vi "Main.vi"() -> ()   [LabVIEW 2018] (continued)
            n437 = call "S7_Read.vi"("TCP"=w5185, "DB #"=u16 20, "读取长度"=u16 1, "寄存器类型"=w5227, "起始地址"=u32 0, "数据类型"=w5225, "error in"=w5184) -> ("TCP"=w5208:refnum<k5>, "数据"=w5222:u32[], "error out"=w5207:errorcluster)  [unwired: 5 in, 1 out]
            n438 = Index Array(array=w5222, index=0 ("索引")) -> (element=w5220:u32)
            n439 = Number To Boolean Array(number=w5220) -> (Boolean array=w5219:bool[])
            n440 = Index Array(array=w5219, index=2 ("索引")) -> (element=w5209:bool)
            "ST502扫码请求" <- w5209
            n441 = Unbundle By Name(w5187) -> ("扫码超时2"=w5200:string)
            n442 = Not Equal?(x=w5200, y="999") -> (x != y?=w5202:bool)
            n443 = Not(x=w5202) -> (.not. x?=w5203:bool)
            n444 = call <vilib>:"Boolean Crossing PtByPt.vi"("direction"=enum16{"either", "false-true", "true-false"}."false-true", "input"=w5209) -> ("crossing"=w5215:bool)  [unwired: 1 in]
            n445 = call <vilib>:"Boolean Crossing PtByPt.vi"("direction"=enum16{"either", "false-true", "true-false"}."true-false", "input"=w5209) -> ("crossing"=w5214:bool)  [unwired: 1 in]
            n446 = call "已用时间13"("Reset"=w5203) -> ("Time has Elapsed"=w5204:bool)  [unwired: 11 in, 7 out]
            n447 = Insert Into Array(array=bool[] [] ("数组"), index=0 ("索引"), new element #1=w5215, new element #2=w5214) -> (w5211:bool[])
            n448 = Boolean Array To Number(Boolean array=w5211) -> (number=w5210:u32)
            n449 = case shown="0, 默认" w5210 {
              tunnel: [cluster{"Data":string[], "State":T1} {"Data"=[], "State"=enum."读数据保存请求2"} ("元素") w5235 w5237] -> w5206
              tunnel: w5199 -> [_ w5236 w5238]
              frame 0, Default {
              }
              frame 1 {
                w5235 = cluster{"Data":string[], "State":T1} {"Data"=[], "State"=enum."读二维码2"} ("元素")
                n450 = Enqueue Element(queue=w5236, element=w5235, timeout in ms (-1)=10 ("超时毫秒(-1)")) -> ()  [unwired: 1 in, 3 out]
              }
              frame 2 {
                w5237 = cluster{"Data":string[], "State":T1} {"Data"=["999"], "State"=enum."扫码回复2"} ("元素")
                n451 = Enqueue Element(queue=w5238, element=w5237, timeout in ms (-1)=10 ("超时毫秒(-1)")) -> ()  [unwired: 1 in, 3 out]
              }
            }
            n452 = case shown="真" w5204 {
              tunnel: w5199 -> [_ w5231]
              frame False {
              }
              frame True {
                n453 = Enqueue Element(queue=w5231, element=cluster{"Data":string[], "State":T1} {"Data"=["999"], "State"=enum."扫码回复2"} ("元素"), timeout in ms (-1)=10 ("超时毫秒(-1)")) -> ()  [unwired: 1 in, 3 out]
              }
            }
          }
          frame "读二维码2" {
            w5255 = u16 0 items=["byte", "word", "Dword"] ("数据类型")
            w5252 = u8 132 items=["I/O (P)"=128, "Input (I)"=129, "Output (Q)"=130, "Bit Memory (M)"=131, "Data (DB)"=132, "Instance Data (DI)"=133, "Local Data (L)"=134, "Predecessor Local Data (VL)"=135] ("寄存器类型")
            n454 = call "S7_Read.vi"("TCP"=w5251, "DB #"=u16 20, "读取长度"=u16 17, "寄存器类型"=w5252, "起始地址"=u32 42, "数据类型"=w5255) -> ("TCP"=w5250:refnum<k5>, "数据"=w5256:u32[], "error out"=w5258:errorcluster)  [unwired: 6 in, 1 out]
            n455 = To Unsigned Word Integer(number=w5256) -> (unsigned 16bit integer=w5257:u16[])
            n456 = call "还原为字符串.vi"("error in (no error)"=w5258, "输入数组"=w5257) -> ("error out"=w5242:errorcluster, "字符串"=w5243:string)  [unwired: 8 in]
            n457 = Match Pattern(string=w5243, regular expression=" " ("正则表达式")) -> (before substring=w5240:string)  [unwired: 1 in, 3 out]
            n458 = flat-sequence {
              tunnel: w5242 -> [w5260]
              tunnel: [w5260] -> w5241
              tunnel: w5240 -> [w5259]
              tunnel: [w5262] -> w5247
              tunnel: w5241 -> [w5261]
              frame #0 {
                "503二维码" <- w5259
              }
              frame #1 {
                n459 = property on="ST503扫码请求(事件)" class="Bool (严格)"(error in=w5261, "Val(Sgnl)"=TRUE ("值(信号)")) -> (error out=w5262:errorcluster)  [unwired: 1 in, 1 out]
              }
            }
          }
          frame "扫码回复2" {
            n460 = Array Size(array=w5272) -> (size(s)=w5273:i32)
            n461 = case shown="3, 默认" w5273 {
              tunnel: w5272 -> [w5298 w5307]
              tunnel: w5271 -> [w5285 w5308]
              tunnel: [w5276 w5310] -> w5270
              tunnel: [w5275 w5309] -> w5269
              tunnel: [w5274 w5306] -> w5264
              frame 3, Default {
                w5288 = u8 132 items=["I/O (P)"=128, "Input (I)"=129, "Output (Q)"=130, "Bit Memory (M)"=131, "Data (DB)"=132, "Instance Data (DI)"=133, "Local Data (L)"=134, "Predecessor Local Data (VL)"=135] ("寄存器类型")
                w5287 = u16 1 items=["byte", "word", "Dword"] ("数据类型")
                w5295 = u8 132 items=["I/O (P)"=128, "Input (I)"=129, "Output (Q)"=130, "Bit Memory (M)"=131, "Data (DB)"=132, "Instance Data (DI)"=133, "Local Data (L)"=134, "Predecessor Local Data (VL)"=135] ("寄存器类型")
                w5296 = u16 1 items=["byte", "word", "Dword"] ("数据类型")
                w5302 = u8 132 items=["I/O (P)"=128, "Input (I)"=129, "Output (Q)"=130, "Bit Memory (M)"=131, "Data (DB)"=132, "Instance Data (DI)"=133, "Local Data (L)"=134, "Predecessor Local Data (VL)"=135] ("寄存器类型")
                w5301 = u16 1 items=["byte", "word", "Dword"] ("数据类型")
                n462 = Index Array(array=w5298) -> (element #1=w5274:string, element #2=w5281:string, element #3=w5280:string)  [unwired: 3 in]
                n463 = Equal?(x=w5280, y="OK") -> (x = y?=w5278:bool)
                n464 = Decimal String To Number(string=w5281, default (0L)=u32 0 ("默认(0 I32)")) -> (number=w5282:u32)  [unwired: 1 in, 1 out]
                n465 = case shown="假" w5278 {
                  tunnel: [u32 2 ("写入数据") u32 1 ("写入数据")] -> w5277
                  frame False {
                  }
                  frame True {
                  }
                }
                n466 = call "S7_Write.vi"("TCP"=w5285, "寄存器类型"=w5302, "DB #"=u16 20, "写入地址"=u32 18, "数据类型"=w5301, "写入数据"=w5282) -> ("TCP"=w5292:refnum<k5>, "error out"=w5293:errorcluster)  [unwired: 7 in, 1 out]
                n467 = call "S7_Write.vi"("TCP"=w5292, "寄存器类型"=w5295, "DB #"=u16 20, "写入地址"=u32 20, "数据类型"=w5296, "写入数据"=w5277, "error in"=w5293) -> ("TCP"=w5284:refnum<k5>, "error out"=w5283:errorcluster)  [unwired: 6 in, 1 out]
                n468 = Decimal String To Number(string=w5274, default (0L)=u32 0 ("默认(0 I32)")) -> (number=w5291:u32)  [unwired: 1 in, 1 out]
                n469 = call "S7_Write.vi"("TCP"=w5284, "寄存器类型"=w5288, "DB #"=u16 20, "写入地址"=u32 14, "数据类型"=w5287, "写入数据"=w5291, "error in"=w5283) -> ("TCP"=w5276:refnum<k5>, "error out"=w5275:errorcluster)  [unwired: 6 in, 1 out]
              }
              frame 1 {
                w5313 = u8 132 items=["I/O (P)"=128, "Input (I)"=129, "Output (Q)"=130, "Bit Memory (M)"=131, "Data (DB)"=132, "Instance Data (DI)"=133, "Local Data (L)"=134, "Predecessor Local Data (VL)"=135] ("寄存器类型")
                w5312 = u16 1 items=["byte", "word", "Dword"] ("数据类型")
                n470 = Index Array(array=w5307) -> (element=w5306:string)  [unwired: 1 in]
                n471 = Decimal String To Number(string=w5306, default (0L)=u32 0 ("默认(0 I32)")) -> (number=w5316:u32)  [unwired: 1 in, 1 out]
                n472 = call "S7_Write.vi"("TCP"=w5308, "寄存器类型"=w5313, "DB #"=u16 20, "写入地址"=u32 14, "数据类型"=w5312, "写入数据"=w5316) -> ("TCP"=w5310:refnum<k5>, "error out"=w5309:errorcluster)  [unwired: 7 in, 1 out]
              }
            }
            "扫码请求回复502" <- w5264
            n473 = Bundle By Name(cluster=w5266, "扫码超时2"=w5264) -> (w5265:T7)
          }
          frame "-- --------------" {
          }
          frame "读数据保存请求2" {
            w5350 = u16 0 items=["byte", "word", "Dword"] ("数据类型")
            w5352 = u8 132 items=["I/O (P)"=128, "Input (I)"=129, "Output (Q)"=130, "Bit Memory (M)"=131, "Data (DB)"=132, "Instance Data (DI)"=133, "Local Data (L)"=134, "Predecessor Local Data (VL)"=135] ("寄存器类型")
            n474 = call "S7_Read.vi"("TCP"=w5333, "DB #"=u16 20, "读取长度"=u16 1, "寄存器类型"=w5352, "起始地址"=u32 0, "数据类型"=w5350) -> ("TCP"=w5332:refnum<k5>, "数据"=w5347:u32[], "error out"=w5331:errorcluster)  [unwired: 6 in, 1 out]
            n475 = Index Array(array=w5347, index=0 ("索引")) -> (element=w5345:u32)
            n476 = Number To Boolean Array(number=w5345) -> (Boolean array=w5344:bool[])
            n477 = Unbundle By Name(w5323) -> ("数据保存超时2"=w5324:string)
            n478 = Index Array(array=w5344, index=3 ("索引")) -> (element=w5334:bool)
            "ST502数据读取" <- w5334
            n479 = Not Equal?(x=w5324, y="999") -> (x != y?=w5326:bool)
            n480 = Not(x=w5326) -> (.not. x?=w5327:bool)
            n481 = call <vilib>:"Boolean Crossing PtByPt.vi"("direction"=enum16{"either", "false-true", "true-false"}."false-true", "input"=w5334) -> ("crossing"=w5337:bool)  [unwired: 1 in]
            n482 = call <vilib>:"Boolean Crossing PtByPt.vi"("direction"=enum16{"either", "false-true", "true-false"}."true-false", "input"=w5334) -> ("crossing"=w5338:bool)  [unwired: 1 in]
            n483 = call "已用时间14"("Reset"=w5327) -> ("Time has Elapsed"=w5328:bool)  [unwired: 11 in, 7 out]
            n484 = Insert Into Array(array=bool[] [] ("数组"), index=0 ("索引"), new element #1=w5337, new element #2=w5338) -> (w5341:bool[])
            n485 = Boolean Array To Number(Boolean array=w5341) -> (number=w5342:u32)
            n486 = case shown="1" w5342 {
              tunnel: [cluster{"Data":string[], "State":T1} {"Data"=[], "State"=enum."看门狗"} ("元素") w5358 w5361] -> w5330
              tunnel: w5322 -> [_ w5359 w5362]
              frame 0, Default {
              }
              frame 1 {
                w5358 = cluster{"Data":string[], "State":T1} {"Data"=[], "State"=enum."读数据2"} ("元素")
                n487 = Enqueue Element(queue=w5359, element=w5358, timeout in ms (-1)=10 ("超时毫秒(-1)")) -> ()  [unwired: 1 in, 3 out]
              }
              frame 2 {
                w5361 = cluster{"Data":string[], "State":T1} {"Data"=["999"], "State"=enum."数据保存回复2"} ("元素")
                n488 = Enqueue Element(queue=w5362, element=w5361, timeout in ms (-1)=10 ("超时毫秒(-1)")) -> ()  [unwired: 1 in, 3 out]
              }
            }
            n489 = case shown="真" w5328 {
              tunnel: w5322 -> [_ w5354]
              frame False {
              }
              frame True {
                n490 = Enqueue Element(queue=w5354, element=cluster{"Data":string[], "State":T1} {"Data"=["999"], "State"=enum."数据保存回复2"} ("元素"), timeout in ms (-1)=10 ("超时毫秒(-1)")) -> ()  [unwired: 1 in, 3 out]
              }
            }
          }
          frame "读数据2" {
            w5373 = u16 1 items=["byte", "word", "Dword"] ("数据类型")
            w5377 = u8 132 items=["I/O (P)"=128, "Input (I)"=129, "Output (Q)"=130, "Bit Memory (M)"=131, "Data (DB)"=132, "Instance Data (DI)"=133, "Local Data (L)"=134, "Predecessor Local Data (VL)"=135] ("寄存器类型")
            n491 = call "S7_Read.vi"("TCP"=w5368, "DB #"=u16 20, "读取长度"=u16 1, "寄存器类型"=w5377, "起始地址"=u32 12, "数据类型"=w5373) -> ("TCP"=w5366:refnum<k5>, "数据"=w5372:u32[], "error out"=w5365:errorcluster)  [unwired: 6 in, 1 out]
            n492 = Index Array(array=w5372) -> (element=w5370:u32)  [unwired: 1 in]
            n493 = Equal?(x=w5370, y=u32 1) -> (x = y?=w5384:bool)
            n494 = case shown="假" w5384 {
              tunnel: ["NG" "OK"] -> w5367
              frame False {
              }
              frame True {
              }
            }
            n495 = Format Date/Time String(time format string (%c)="%Y-%m-%d" ("时间格式字符串(%c)")) -> (date/time string=w5379:string)  [unwired: 2 in]
            n496 = Get Date/Time String() -> (time string=w5378:string)  [unwired: 3 in, 1 out]
            n497 = Insert Into Array(array=string[] [] ("数组"), index=0 ("索引"), new element #1="503" ("新元素/子数组"), new element #2=w5367, new element #3=w5379, new element #4=w5378, new element #5=w5367) -> (w5363:string[])
            n498 = flat-sequence {
              tunnel: w5365 -> [w5389]
              tunnel: [w5389] -> w5364
              tunnel: w5363 -> [w5388]
              tunnel: [w5391] -> w5371
              tunnel: w5364 -> [w5390]
              frame #0 {
                "503读取数据" <- w5388
              }
              frame #1 {
                n499 = property on="ST503数据读取（事件）" class="Bool (严格)"(error in=w5390, "Val(Sgnl)"=TRUE ("值(信号)")) -> (error out=w5391:errorcluster)  [unwired: 1 in, 1 out]
              }
            }
          }
          frame "数据保存回复2" {
            w5408 = u8 132 items=["I/O (P)"=128, "Input (I)"=129, "Output (Q)"=130, "Bit Memory (M)"=131, "Data (DB)"=132, "Instance Data (DI)"=133, "Local Data (L)"=134, "Predecessor Local Data (VL)"=135] ("寄存器类型")
            w5409 = u16 1 items=["byte", "word", "Dword"] ("数据类型")
            n500 = Index Array(array=w5402, index=0 ("索引")) -> (element=w5395:string)
            "数据保存请求回复502" <- w5395
            n501 = Decimal String To Number(string=w5395, default (0L)=u32 0 ("默认(0 I32)")) -> (number=w5404:u32)  [unwired: 1 in, 1 out]
            n502 = call "S7_Write.vi"("TCP"=w5403, "寄存器类型"=w5408, "DB #"=u16 20, "写入地址"=u32 16, "数据类型"=w5409, "写入数据"=w5404) -> ("TCP"=w5401:refnum<k5>, "error out"=w5400:errorcluster)  [unwired: 7 in, 1 out]
            n503 = Bundle By Name(cluster=w5397, "数据保存超时2"=w5395) -> (w5396:T7)
          }
          frame "------------" {
          }
          frame "看门狗" {
            w5426 = "\r" ("正则表达式")
            w5435 = u16 0 items=["byte", "word", "Dword"] ("数据类型")
            w5437 = u8 132 items=["I/O (P)"=128, "Input (I)"=129, "Output (Q)"=130, "Bit Memory (M)"=131, "Data (DB)"=132, "Instance Data (DI)"=133, "Local Data (L)"=134, "Predecessor Local Data (VL)"=135] ("寄存器类型")
            w5458 = u8 132 items=["I/O (P)"=128, "Input (I)"=129, "Output (Q)"=130, "Bit Memory (M)"=131, "Data (DB)"=132, "Instance Data (DI)"=133, "Local Data (L)"=134, "Predecessor Local Data (VL)"=135] ("寄存器类型")
            w5457 = u16 1 items=["byte", "word", "Dword"] ("数据类型")
            n504 = Unbundle By Name(w5446) -> ("看门狗"=w5455:string)
            n505 = Decimal String To Number(string=w5455) -> (number=w5454:i32)  [unwired: 2 in, 1 out]
            n506 = Equal?(x=w5454, y=0) -> (x = y?=w5452:bool)
            n507 = case shown="假" w5452 {
              tunnel: [0 ("y") 1 ("y")] -> w5447
              frame False {
              }
              frame True {
              }
            }
            "50" <- w5447
            n508 = call "S7_Write.vi"("TCP"=w5451, "寄存器类型"=w5458, "DB #"=u16 20, "写入地址"=u32 22, "数据类型"=w5457, "写入数据"=w5447) -> ("TCP"=w5433:refnum<k5>, "error out"=w5432:errorcluster)  [unwired: 7 in, 1 out]
            n509 = Number To Decimal String(number=w5447) -> (decimal integer string=w5448:string)  [unwired: 1 in]
            n510 = Bundle By Name(cluster=w5446, "看门狗"=w5448) -> (w5445:T7)
            n511 = call "S7_Read.vi"("TCP"=w5433, "DB #"=u16 20, "读取长度"=u16 100, "寄存器类型"=w5437, "起始地址"=u32 60, "数据类型"=w5435, "error in"=w5432) -> ("TCP"=w5421:refnum<k5>, "数据"=w5443:u32[], "error out"=w5419:errorcluster)  [unwired: 5 in, 1 out]
            n512 = To Unsigned Word Integer(number=w5443) -> (unsigned 16bit integer=w5444:u16[])
            n513 = call "还原为字符串.vi"("输入数组"=w5444) -> ("字符串"=w5442:string)  [unwired: 9 in, 1 out]
            n514 = for {
              N: 5 -> [_]
              tunnel: w5442 -> [w5478]
              tunnel: [w5477] -> w5434 mode=indexing
              shift-right: [w5473] -> _
              shift-left: 0 ("长度（剩余）") -> [w5475]
              n515 = String Subset(string=w5478, offset (0)=w5475, length (rest)=20 ("长度（剩余）")) -> (substring=w5477:string)
              n516 = Add(x=w5475, y=20) -> (x+y=w5473:i32)
            }
            n517 = Index Array(array=w5434) -> (element #1=w5431:string, element #2=w5430:string, element #3=w5429:string, element #4=w5428:string, element #5=w5427:string)  [unwired: 5 in]
            n518 = Match Pattern(string=w5431, regular expression=w5426) -> (before substring=w5417:string)  [unwired: 1 in, 3 out]
            n519 = Match Pattern(string=w5430, regular expression=w5426) -> (before substring=→"ST502 Form Seal 5026860":string)  [unwired: 1 in, 3 out]
            n520 = Match Pattern(string=w5429, regular expression=w5426) -> (before substring=→"ST502 Support Ring 5027083":string)  [unwired: 1 in, 3 out]
            n521 = Match Pattern(string=w5428, regular expression=w5426) -> (before substring=→"ST502 O-Ring M0104976":string)  [unwired: 1 in, 3 out]
            n522 = Match Pattern(string=w5427, regular expression=w5426) -> (before substring=→"ST502 Pressure Plate M0105053":string)  [unwired: 1 in, 3 out]
            n523 = disable-structure shown="启用" {
              disable-tunnel: w5421 -> [w5462 w5466]
              disable-tunnel: [w5462 w5469] -> w5420
              disable-tunnel: w5419 -> [w5463 w5467]
              disable-tunnel: [w5463 w5468] -> w5418
              frame Disabled {
              }
              frame Enabled {
                w5471 = u8 132 items=["I/O (P)"=128, "Input (I)"=129, "Output (Q)"=130, "Bit Memory (M)"=131, "Data (DB)"=132, "Instance Data (DI)"=133, "Local Data (L)"=134, "Predecessor Local Data (VL)"=135] ("寄存器类型")
                w5465 = u16 1 items=["byte", "word", "Dword"] ("数据类型")
                n524 = local read "80产品型号"() -> (w5464:u32)
                n525 = call "S7_Write.vi"("TCP"=w5466, "寄存器类型"=w5471, "DB #"=u16 20, "写入地址"=u32 188, "数据类型"=w5465, "写入数据"=w5464, "error in"=w5467) -> ("TCP"=w5469:refnum<k5>, "error out"=w5468:errorcluster)  [unwired: 6 in, 1 out]
              }
            }
            n526 = disable-structure shown="启用" {
              disable-tunnel: w5417 -> [w5460 _]
              disable-tunnel: [w5460 "20181017/148"] -> w5416
              frame Disabled {
              }
              frame Enabled {
              }
            }
            "ST40 Circlip 5026621" <- w5416
          }
        }
      }
      n527 = while {
        shift-right: [w5486] -> _
        shift-left: cluster{"Data":string[], "State":T1} {"Data"=[], "State"=enum."PLC通讯初始化"} ("元素") -> [w5487]
        shift-right: [w5495] -> _
        shift-left: w133 -> [w5492]
        shift-right: [w5496] -> _
        shift-left: _ -> [w5493]
        tunnel: w115 -> [w5488]
        tunnel: w114 -> [w5483]
        tunnel: w132 -> [_]
        shift-right: [w5482] -> _
        shift-left: _ -> [w5481]
        stop <- w5484 stop-if-true
        # "OP60"
        n528 = local read "退出"() -> (w5491:bool)
        n529 = Wait (ms)(milliseconds to wait=u32 20 ("等待时间（毫秒）")) -> ()  [unwired: 1 out]
        n530 = call "状态判断.vi"("error IO"=w5492, "退出？"=w5491, "簇 输入"=w5487, "队列输入"=w5488) -> ("簇"=w5490:cluster{"Data":string[], "State":T1})  [unwired: 6 in, 1 out]
        n531 = Unbundle By Name(w5490) -> ("Data"=w5485:string[], "State"=w5489:T1)
        "60_State" <- w5489
        n532 = case shown="\"看门狗\"" w5489 {
          tunnel: [w5504 w5545 w5567 w5598 w5619 w5670 w5690 w5722 w5749 w5764 refnum<k5> refnum ("TCP") refnum<k5> refnum ("TCP") w5786 w5811 w5852 w5873 w5924 w5935 w5975 w6005 w6014] -> w5496
          tunnel: [w5503 errorcluster {"status"=FALSE, "code"=0, "source"=""} ("error out") w5566 w5594 w5618 errorcluster {"status"=FALSE, "code"=0, "source"=""} ("error out") w5689 w5712 w5750 errorcluster {"status"=FALSE, "code"=0, "source"=""} ("error out") errorcluster {"status"=FALSE, "code"=0, "source"=""} ("error out") w5776 errorcluster {"status"=FALSE, "code"=0, "source"=""} ("error out") w5808 w5851 w5872 errorcluster {"status"=FALSE, "code"=0, "source"=""} ("error out") w5934 w5974 w6004 w6016] -> w5495
          tunnel: w5493 -> [_ w5545 w5568 w5599 w5620 w5670 w5691 w5736 w5752 w5764 w5770 w5777 w5786 w5792 w5853 w5874 w5924 w5936 w5970 w6006 w6046]
          tunnel: w5488 -> [w5531 _ w5548 _ _ _ w5671 _ _ _ w5766 w5778 _ w5802 _ _ _ w5925 _ _ _]
          tunnel: [cluster{"Data":string[], "State":T1} {"Data"=[], "State"=enum."读扫码请求"} ("元素") cluster{"Data":string[], "State":T1} {"Data"=[], "State"=enum."读扫码请求"} ("元素") w5556 cluster{"Data":string[], "State":T1} {"Data"=[], "State"=enum."读数据保存请求"} ("元素") cluster{"Data":string[], "State":T1} {"Data"=[], "State"=enum."读数据保存请求"} ("元素") cluster{"Data":string[], "State":T1} {"Data"=[], "State"=enum."读数据保存请求"} ("元素") w5679 cluster{"Data":string[], "State":T1} {"Data"=[], "State"=enum."读扫码请求2"} ("元素") cluster{"Data":string[], "State":T1} {"Data"=[], "State"=enum."读扫码请求2"} ("元素") cluster{"Data":string[], "State":T1} {"Data"=[], "State"=enum."读扫码请求2"} ("元素") cluster{"Data":string[], "State":T1} {"Data"=[], "State"=enum."PLC通讯初始化"} ("元素") cluster{"Data":string[], "State":T1} {"Data"=[], "State"=enum."退出"} ("元素") cluster{"Data":string[], "State":T1} {"Data"=[], "State"=enum."读扫码请求2"} ("元素") w5810 cluster{"Data":string[], "State":T1} {"Data"=[], "State"=enum."读数据保存请求2"} ("元素") cluster{"Data":string[], "State":T1} {"Data"=[], "State"=enum."读数据保存请求2"} ("元素") cluster{"Data":string[], "State":T1} {"Data"=[], "State"=enum."读数据保存请求2"} ("元素") w5933 cluster{"Data":string[], "State":T1} {"Data"=[], "State"=enum."看门狗"} ("元素") cluster{"Data":string[], "State":T1} {"Data"=[], "State"=enum."看门狗"} ("元素") cluster{"Data":string[], "State":T1} {"Data"=[], "State"=enum."读扫码请求"} ("元素")] -> w5486
          tunnel: w5485 -> [_ _ _ _ w5616 _ _ _ w5751 _ _ _ _ _ _ w5875 _ _ _ w6003 _]
          tunnel: [FALSE FALSE FALSE FALSE FALSE FALSE FALSE FALSE FALSE FALSE FALSE TRUE FALSE FALSE FALSE FALSE FALSE FALSE FALSE FALSE FALSE] -> w5484
          tunnel: w5483 -> [_ _ _ _ _ _ _ w5729 _ _ w5767 w5779 _ _ _ _ _ _ _ _ _]
          tunnel: [T9 {"扫码超时1"="999", "数据保存超时1"="999", "扫码超时2"="999", "数据保存超时2"="999", "看门狗"="999"} w5541 w5549 w5595 w5614 w5666 w5672 w5719 w5745 w5760 w5765 w5774 w5782 w5790 w5848 w5868 w5920 w5926 w5971 w5998 w6040] -> w5482
          tunnel: w5481 -> [_ w5541 w5549 w5595 w5615 w5666 w5672 w5719 w5746 w5760 w5765 w5774 w5782 w5791 w5848 w5869 w5920 w5926 w5971 w6000 w6041]
          frame "PLC通讯初始化", Default {
            w5516 = u16 0 items=["byte", "word", "Dword"] ("数据类型")
            w5520 = u8 132 items=["I/O (P)"=128, "Input (I)"=129, "Output (Q)"=130, "Bit Memory (M)"=131, "Data (DB)"=132, "Instance Data (DI)"=133, "Local Data (L)"=134, "Predecessor Local Data (VL)"=135] ("寄存器类型")
            w5509 = u16 0 items=["byte", "word", "Dword"] ("数据类型")
            w5513 = u8 132 items=["I/O (P)"=128, "Input (I)"=129, "Output (Q)"=130, "Bit Memory (M)"=131, "Data (DB)"=132, "Instance Data (DI)"=133, "Local Data (L)"=134, "Predecessor Local Data (VL)"=135] ("寄存器类型")
            w5539 = u8 0 items=["S7-1200.200.200SMART"=0, "S7-300"=2, "S7-400"=3] ("PLC 系列")
            n533 = call "S7_Open.vi"("IP 地址"="192.168.0.60", "PLC 系列"=w5539, "超时（MS）"=100) -> ("TCP"=w5506:refnum<k5>, "error out"=w5505:errorcluster)  [unwired: 10 in, 1 out]
            n534 = Unbundle By Name(w5505) -> ("status"=→"ST60通讯状态":bool)
            n535 = Enqueue Element(queue=w5531, element=cluster{"Data":string[], "State":T1} {"Data"=["999"], "State"=enum."扫码回复"} ("元素")) -> (queue out=w5535:refnum<queue>, error out=w5534:errorcluster)  [unwired: 2 in, 1 out]
            n536 = call "S7_Read.vi"("TCP"=w5506, "DB #"=u16 20, "读取长度"=u16 17, "寄存器类型"=w5513, "起始地址"=u32 24, "数据类型"=w5509, "error in"=w5505) -> ("TCP"=w5521:refnum<k5>, "数据"=w5508:u32[], "error out"=w5522:errorcluster)  [unwired: 5 in, 1 out]
            n537 = To Unsigned Word Integer(number=w5508) -> (unsigned 16bit integer=w5507:u16[])
            n538 = call "还原为字符串.vi"("输入数组"=w5507) -> ("字符串"=w5501:string)  [unwired: 9 in, 1 out]
            n539 = Enqueue Element(queue=w5535, element=cluster{"Data":string[], "State":T1} {"Data"=["999"], "State"=enum."数据保存回复"} ("元素"), error in (no error)=w5534) -> (queue out=w5524:refnum<queue>, error out=w5523:errorcluster)  [unwired: 1 in, 1 out]
            n540 = Match Pattern(string=w5501, regular expression=" " ("正则表达式")) -> (before substring=w5500:string)  [unwired: 1 in, 3 out]
            n541 = local write "601二维码"(w5500) -> ()
            n542 = Enqueue Element(queue=w5524, element=cluster{"Data":string[], "State":T1} {"Data"=["999"], "State"=enum."扫码回复2"} ("元素"), error in (no error)=w5523) -> (queue out=w5527:refnum<queue>, error out=w5528:errorcluster)  [unwired: 1 in, 1 out]
            n543 = call "S7_Read.vi"("TCP"=w5521, "DB #"=u16 20, "读取长度"=u16 17, "寄存器类型"=w5520, "起始地址"=u32 42, "数据类型"=w5516, "error in"=w5522) -> ("TCP"=w5504:refnum<k5>, "数据"=w5515:u32[], "error out"=w5503:errorcluster)  [unwired: 5 in, 1 out]
            n544 = Enqueue Element(queue=w5527, element=cluster{"Data":string[], "State":T1} {"Data"=["999"], "State"=enum."数据保存回复2"} ("元素"), error in (no error)=w5528) -> ()  [unwired: 1 in, 3 out]
            n545 = To Unsigned Word Integer(number=w5515) -> (unsigned 16bit integer=w5514:u16[])
            n546 = call "还原为字符串.vi"("输入数组"=w5514) -> ("字符串"=w5498:string)  [unwired: 9 in, 1 out]
            n547 = Match Pattern(string=w5498, regular expression=" " ("正则表达式")) -> (before substring=w5497:string)  [unwired: 1 in, 3 out]
            n548 = local write "602二维码"(w5497) -> ()
          }
          frame "--------------" {
          }
          frame "读扫码请求" {
            w5576 = u16 0 items=["byte", "word", "Dword"] ("数据类型")
            w5578 = u8 132 items=["I/O (P)"=128, "Input (I)"=129, "Output (Q)"=130, "Bit Memory (M)"=131, "Data (DB)"=132, "Instance Data (DI)"=133, "Local Data (L)"=134, "Predecessor Local Data (VL)"=135] ("寄存器类型")
            n549 = call "S7_Read.vi"("TCP"=w5568, "DB #"=u16 20, "读取长度"=u16 1, "寄存器类型"=w5578, "起始地址"=u32 0, "数据类型"=w5576) -> ("TCP"=w5567:refnum<k5>, "数据"=w5573:u32[], "读取成功"=w5546:bool, "error out"=w5566:errorcluster)  [unwired: 6 in]
            n550 = Not(x=w5546) -> (.not. x?=w5547:bool)
            n551 = local write "ST60通讯状态"(w5547) -> ()
            n552 = Index Array(array=w5573, index=0 ("索引")) -> (element=w5571:u32)
            n553 = Number To Boolean Array(number=w5571) -> (Boolean array=w5570:bool[])
            n554 = Index Array(array=w5570, index=0 ("索引")) -> (element=w5555:bool)
            "ST601扫码请求" <- w5555
            n555 = Unbundle By Name(w5549) -> ("扫码超时1"=w5550:string)
            n556 = Not Equal?(x=w5550, y="999") -> (x != y?=w5552:bool)
            n557 = Not(x=w5552) -> (.not. x?=w5553:bool)
            n558 = call <vilib>:"Boolean Crossing PtByPt.vi"("direction"=enum16{"either", "false-true", "true-false"}."false-true", "input"=w5555) -> ("crossing"=w5562:bool)  [unwired: 1 in]
            n559 = call <vilib>:"Boolean Crossing PtByPt.vi"("direction"=enum16{"either", "false-true", "true-false"}."true-false", "input"=w5555) -> ("crossing"=w5561:bool)  [unwired: 1 in]
            n560 = call "已用时间17"("Reset"=w5553) -> ("Time has Elapsed"=w5554:bool)  [unwired: 11 in, 7 out]
            n561 = Insert Into Array(array=bool[] [] ("数组"), index=0 ("索引"), new element #1=w5562, new element #2=w5561) -> (w5558:bool[])
            n562 = Boolean Array To Number(Boolean array=w5558) -> (number=w5557:u32)
            n563 = case shown="2" w5557 {
              tunnel: [cluster{"Data":string[], "State":T1} {"Data"=[], "State"=enum."读数据保存请求"} ("元素") w5584 w5587] -> w5556
              tunnel: w5548 -> [_ w5585 w5588]
              frame 0, Default {
              }
              frame 1 {
                w5584 = cluster{"Data":string[], "State":T1} {"Data"=[], "State"=enum."读二维码"} ("元素")
                n564 = Enqueue Element(queue=w5585, element=w5584, timeout in ms (-1)=10 ("超时毫秒(-1)")) -> ()  [unwired: 1 in, 3 out]
              }
              frame 2 {
                w5587 = cluster{"Data":string[], "State":T1} {"Data"=["999"], "State"=enum."扫码回复"} ("元素")
                n565 = Enqueue Element(queue=w5588, element=w5587, timeout in ms (-1)=10 ("超时毫秒(-1)")) -> ()  [unwired: 1 in, 3 out]
              }
            }
            n566 = case shown="真" w5554 {
              tunnel: w5548 -> [_ w5580]
              frame False {
              }
              frame True {
                n567 = Enqueue Element(queue=w5580, element=cluster{"Data":string[], "State":T1} {"Data"=["999"], "State"=enum."扫码回复"} ("元素"), timeout in ms (-1)=10 ("超时毫秒(-1)")) -> ()  [unwired: 1 in, 3 out]
              }
            }
          }
          frame "读二维码" {
            w5604 = u16 0 items=["byte", "word", "Dword"] ("数据类型")
            w5600 = u8 132 items=["I/O (P)"=128, "Input (I)"=129, "Output (Q)"=130, "Bit Memory (M)"=131, "Data (DB)"=132, "Instance Data (DI)"=133, "Local Data (L)"=134, "Predecessor Local Data (VL)"=135] ("寄存器类型")
            n568 = call "S7_Read.vi"("TCP"=w5599, "DB #"=u16 20, "读取长度"=u16 17, "寄存器类型"=w5600, "起始地址"=u32 24, "数据类型"=w5604) -> ("TCP"=w5598:refnum<k5>, "数据"=w5605:u32[], "error out"=w5607:errorcluster)  [unwired: 6 in, 1 out]
            n569 = To Unsigned Word Integer(number=w5605) -> (unsigned 16bit integer=w5606:u16[])
            n570 = call "还原为字符串.vi"("error in (no error)"=w5607, "输入数组"=w5606) -> ("error out"=w5591:errorcluster, "字符串"=w5592:string)  [unwired: 8 in]
            n571 = Match Pattern(string=w5592, regular expression=" " ("正则表达式")) -> (before substring=w5589:string)  [unwired: 1 in, 3 out]
            n572 = flat-sequence {
              tunnel: w5591 -> [w5609]
              tunnel: [w5609] -> w5590
              tunnel: w5589 -> [w5608]
              tunnel: [w5611] -> w5594
              tunnel: w5590 -> [w5610]
              frame #0 {
                "601二维码" <- w5608
              }
              frame #1 {
                n573 = property on="ST601扫码请求(事件)" class="Bool (严格)"(error in=w5610, "Val(Sgnl)"=TRUE ("值(信号)")) -> (error out=w5611:errorcluster)  [unwired: 1 in, 1 out]
              }
            }
          }
          frame "扫码回复" {
            n574 = Array Size(array=w5616) -> (size(s)=w5617:i32)
            n575 = case shown="3, 默认" w5617 {
              tunnel: w5616 -> [w5624 w5658]
              tunnel: w5620 -> [w5625 w5645]
              tunnel: [w5627 w5636] -> w5619
              tunnel: [w5626 w5635] -> w5618
              tunnel: [w5623 w5634] -> w5613
              frame 1 {
                w5630 = u8 132 items=["I/O (P)"=128, "Input (I)"=129, "Output (Q)"=130, "Bit Memory (M)"=131, "Data (DB)"=132, "Instance Data (DI)"=133, "Local Data (L)"=134, "Predecessor Local Data (VL)"=135] ("寄存器类型")
                w5629 = u16 1 items=["byte", "word", "Dword"] ("数据类型")
                n576 = Index Array(array=w5624) -> (element=w5623:string)  [unwired: 1 in]
                n577 = Decimal String To Number(string=w5623, default (0L)=u32 0 ("默认(0 I32)")) -> (number=w5633:u32)  [unwired: 1 in, 1 out]
                n578 = call "S7_Write.vi"("TCP"=w5625, "寄存器类型"=w5630, "DB #"=u16 20, "写入地址"=u32 2, "数据类型"=w5629, "写入数据"=w5633) -> ("TCP"=w5627:refnum<k5>, "error out"=w5626:errorcluster)  [unwired: 7 in, 1 out]
              }
              frame 3, Default {
                w5648 = u8 132 items=["I/O (P)"=128, "Input (I)"=129, "Output (Q)"=130, "Bit Memory (M)"=131, "Data (DB)"=132, "Instance Data (DI)"=133, "Local Data (L)"=134, "Predecessor Local Data (VL)"=135] ("寄存器类型")
                w5647 = u16 1 items=["byte", "word", "Dword"] ("数据类型")
                w5655 = u8 132 items=["I/O (P)"=128, "Input (I)"=129, "Output (Q)"=130, "Bit Memory (M)"=131, "Data (DB)"=132, "Instance Data (DI)"=133, "Local Data (L)"=134, "Predecessor Local Data (VL)"=135] ("寄存器类型")
                w5656 = u16 1 items=["byte", "word", "Dword"] ("数据类型")
                w5662 = u8 132 items=["I/O (P)"=128, "Input (I)"=129, "Output (Q)"=130, "Bit Memory (M)"=131, "Data (DB)"=132, "Instance Data (DI)"=133, "Local Data (L)"=134, "Predecessor Local Data (VL)"=135] ("寄存器类型")
                w5661 = u16 1 items=["byte", "word", "Dword"] ("数据类型")
                n579 = Index Array(array=w5658) -> (element #1=w5634:string, element #2=w5641:string, element #3=w5640:string)  [unwired: 3 in]
                n580 = Equal?(x=w5640, y="OK") -> (x = y?=w5638:bool)
                n581 = Decimal String To Number(string=w5641, default (0L)=u32 0 ("默认(0 I32)")) -> (number=w5642:u32)  [unwired: 1 in, 1 out]
                n582 = case shown="假" w5638 {
                  tunnel: [u32 2 ("写入数据") u32 1 ("写入数据")] -> w5637
                  frame False {
                  }
                  frame True {
                  }
                }
                n583 = call "S7_Write.vi"("TCP"=w5645, "寄存器类型"=w5662, "DB #"=u16 20, "写入地址"=u32 8, "数据类型"=w5661, "写入数据"=w5642) -> ("TCP"=w5652:refnum<k5>, "error out"=w5653:errorcluster)  [unwired: 7 in, 1 out]
                n584 = call "S7_Write.vi"("TCP"=w5652, "寄存器类型"=w5655, "DB #"=u16 20, "写入地址"=u32 10, "数据类型"=w5656, "写入数据"=w5637, "error in"=w5653) -> ("TCP"=w5644:refnum<k5>, "error out"=w5643:errorcluster)  [unwired: 6 in, 1 out]
                n585 = Decimal String To Number(string=w5634, default (0L)=u32 0 ("默认(0 I32)")) -> (number=w5651:u32)  [unwired: 1 in, 1 out]
                n586 = call "S7_Write.vi"("TCP"=w5644, "寄存器类型"=w5648, "DB #"=u16 20, "写入地址"=u32 2, "数据类型"=w5647, "写入数据"=w5651, "error in"=w5643) -> ("TCP"=w5636:refnum<k5>, "error out"=w5635:errorcluster)  [unwired: 6 in, 1 out]
              }
            }
            "扫码请求回复601" <- w5613
            n587 = Bundle By Name(cluster=w5615, "扫码超时1"=w5613) -> (w5614:T9)
          }
          frame "-------------" {
          }
          frame "读数据保存请求" {
            w5699 = u16 0 items=["byte", "word", "Dword"] ("数据类型")
            w5701 = u8 132 items=["I/O (P)"=128, "Input (I)"=129, "Output (Q)"=130, "Bit Memory (M)"=131, "Data (DB)"=132, "Instance Data (DI)"=133, "Local Data (L)"=134, "Predecessor Local Data (VL)"=135] ("寄存器类型")
            n588 = call "S7_Read.vi"("TCP"=w5691, "DB #"=u16 20, "读取长度"=u16 1, "寄存器类型"=w5701, "起始地址"=u32 0, "数据类型"=w5699) -> ("TCP"=w5690:refnum<k5>, "数据"=w5696:u32[], "error out"=w5689:errorcluster)  [unwired: 6 in, 1 out]
            n589 = Index Array(array=w5696, index=0 ("索引")) -> (element=w5694:u32)
            n590 = Number To Boolean Array(number=w5694) -> (Boolean array=w5693:bool[])
            n591 = Unbundle By Name(w5672) -> ("数据保存超时1"=w5673:string)
            n592 = Index Array(array=w5693, index=1 ("索引")) -> (element=w5678:bool)
            "ST601数据读取" <- w5678
            n593 = Not Equal?(x=w5673, y="999") -> (x != y?=w5675:bool)
            n594 = Not(x=w5675) -> (.not. x?=w5676:bool)
            n595 = call <vilib>:"Boolean Crossing PtByPt.vi"("direction"=enum16{"either", "false-true", "true-false"}."false-true", "input"=w5678) -> ("crossing"=w5682:bool)  [unwired: 1 in]
            n596 = call <vilib>:"Boolean Crossing PtByPt.vi"("direction"=enum16{"either", "false-true", "true-false"}."true-false", "input"=w5678) -> ("crossing"=w5683:bool)  [unwired: 1 in]
            n597 = call "已用时间18"("Reset"=w5676) -> ("Time has Elapsed"=w5677:bool)  [unwired: 11 in, 7 out]
            n598 = Insert Into Array(array=bool[] [] ("数组"), index=0 ("索引"), new element #1=w5682, new element #2=w5683) -> (w5686:bool[])
            n599 = Boolean Array To Number(Boolean array=w5686) -> (number=w5687:u32)
            n600 = case shown="2" w5687 {
              tunnel: [cluster{"Data":string[], "State":T1} {"Data"=[], "State"=enum."读扫码请求2"} ("元素") w5707 w5709] -> w5679
              tunnel: w5671 -> [_ w5708 w5710]
              frame 0, Default {
              }
              frame 1 {
                w5707 = cluster{"Data":string[], "State":T1} {"Data"=[], "State"=enum."读数据"} ("元素")
                n601 = Enqueue Element(queue=w5708, element=w5707, timeout in ms (-1)=10 ("超时毫秒(-1)")) -> ()  [unwired: 1 in, 3 out]
              }
              frame 2 {
                w5709 = cluster{"Data":string[], "State":T1} {"Data"=["999"], "State"=enum."数据保存回复"} ("元素")
                n602 = Enqueue Element(queue=w5710, element=w5709, timeout in ms (-1)=10 ("超时毫秒(-1)")) -> ()  [unwired: 1 in, 3 out]
              }
            }
            n603 = case shown="真" w5677 {
              tunnel: w5671 -> [_ w5703]
              frame False {
              }
              frame True {
                n604 = Enqueue Element(queue=w5703, element=cluster{"Data":string[], "State":T1} {"Data"=["999"], "State"=enum."数据保存回复"} ("元素"), timeout in ms (-1)=10 ("超时毫秒(-1)")) -> ()  [unwired: 1 in, 3 out]
              }
            }
          }
          frame "读数据" {
            w5741 = u16 1 items=["byte", "word", "Dword"] ("数据类型")
            w5737 = u8 132 items=["I/O (P)"=128, "Input (I)"=129, "Output (Q)"=130, "Bit Memory (M)"=131, "Data (DB)"=132, "Instance Data (DI)"=133, "Local Data (L)"=134, "Predecessor Local Data (VL)"=135] ("寄存器类型")
            n605 = call "S7_Read.vi"("TCP"=w5736, "DB #"=u16 20, "读取长度"=u16 1, "寄存器类型"=w5737, "起始地址"=u32 6, "数据类型"=w5741) -> ("TCP"=w5722:refnum<k5>, "数据"=w5733:u32[], "error out"=w5721:errorcluster)  [unwired: 6 in, 1 out]
            n606 = local read "ST60 Disk Spring 5024300"() -> (w5717:string)
            n607 = local read "ST60 Sleeve 5020302"() -> (w5716:string)
            n608 = Index Array(array=w5733) -> (element #1=w5720:u32)  [unwired: 2 in, 1 out]
            n609 = local read "ST60 Eclip 5018568"() -> (w5715:string)
            n610 = Equal?(x=w5720, y=u32 1) -> (x = y?=w5731:bool)
            n611 = case shown="假" w5731 {
              tunnel: ["NG" "OK"] -> w5718
              frame False {
              }
              frame True {
              }
            }
            n612 = Format Date/Time String(time format string (%c)="%Y-%m-%d" ("时间格式字符串(%c)")) -> (date/time string=w5724:string)  [unwired: 2 in]
            n613 = Get Date/Time String() -> (time string=w5723:string)  [unwired: 3 in, 1 out]
            n614 = Insert Into Array(array=string[] [] ("数组"), index=0 ("索引"), new element #1="601" ("新元素/子数组"), new element #2=w5718, new element #3=w5724, new element #4=w5723, new element #5=w5718, new element #6=w5717, new element #7=w5716, new element #8=w5715) -> (w5730:string[])
            n615 = Enqueue Element(queue=w5729, element=w5730, error in (no error)=w5721) -> (error out=w5713:errorcluster)  [unwired: 1 in, 2 out]
            n616 = property on="ST601数据读取（事件）" class="Bool (严格)"(error in=w5713, "Val(Sgnl)"=TRUE ("值(信号)")) -> (error out=w5712:errorcluster)  [unwired: 1 in, 1 out]
          }
          frame "数据保存回复" {
            w5757 = u8 132 items=["I/O (P)"=128, "Input (I)"=129, "Output (Q)"=130, "Bit Memory (M)"=131, "Data (DB)"=132, "Instance Data (DI)"=133, "Local Data (L)"=134, "Predecessor Local Data (VL)"=135] ("寄存器类型")
            w5758 = u16 1 items=["byte", "word", "Dword"] ("数据类型")
            n617 = Index Array(array=w5751, index=0 ("索引")) -> (element=w5744:string)
            "数据保存请求回复601" <- w5744
            n618 = Decimal String To Number(string=w5744, default (0L)=u32 0 ("默认(0 I32)")) -> (number=w5753:u32)  [unwired: 1 in, 1 out]
            n619 = call "S7_Write.vi"("TCP"=w5752, "寄存器类型"=w5757, "DB #"=u16 20, "写入地址"=u32 4, "数据类型"=w5758, "写入数据"=w5753) -> ("TCP"=w5749:refnum<k5>, "error out"=w5750:errorcluster)  [unwired: 7 in, 1 out]
            n620 = Bundle By Name(cluster=w5746, "数据保存超时1"=w5744) -> (w5745:T9)
          }
          frame "-----------------" {
          }
          frame "错误" {
            n621 = Flush Queue(queue=w5767) -> ()  [unwired: 1 in, 3 out]
            n622 = Flush Queue(queue=w5766) -> ()  [unwired: 1 in, 3 out]
            n623 = call "S7_Close.vi"("TCP Connection Ref"=w5770) -> ("error out"=w5768:errorcluster)  [unwired: 10 in]
            n624 = call <vilib>:"Clear Errors.vi"("error in (no error)"=w5768) -> ()  [unwired: 5 in, 2 out]
          }
          frame "退出" {
            n625 = Release Queue(queue=w5779) -> ()  [unwired: 2 in, 3 out]
            n626 = Release Queue(queue=w5778) -> ()  [unwired: 2 in, 3 out]
            n627 = call "S7_Close.vi"("TCP Connection Ref"=w5777) -> ("error out"=w5776:errorcluster)  [unwired: 10 in]
          }
          frame "-------------------" {
          }
          frame "读扫码请求2" {
            w5800 = u8 132 items=["I/O (P)"=128, "Input (I)"=129, "Output (Q)"=130, "Bit Memory (M)"=131, "Data (DB)"=132, "Instance Data (DI)"=133, "Local Data (L)"=134, "Predecessor Local Data (VL)"=135] ("寄存器类型")
            w5799 = u16 1 items=["byte", "word", "Dword"] ("数据类型")
            w5828 = u16 0 items=["byte", "word", "Dword"] ("数据类型")
            w5830 = u8 132 items=["I/O (P)"=128, "Input (I)"=129, "Output (Q)"=130, "Bit Memory (M)"=131, "Data (DB)"=132, "Instance Data (DI)"=133, "Local Data (L)"=134, "Predecessor Local Data (VL)"=135] ("寄存器类型")
            n628 = Unbundle By Name(w5791) -> ("看门狗"=w5797:string)
            n629 = Decimal String To Number(string=w5797) -> (number=w5796:i32)  [unwired: 2 in, 1 out]
            n630 = Equal?(x=w5796, y=0) -> (x = y?=w5794:bool)
            n631 = case shown="假" w5794 {
              tunnel: [0 ("y") 1 ("y")] -> w5787
              frame False {
              }
              frame True {
              }
            }
            n632 = local write "60"(w5787) -> ()
            n633 = Number To Decimal String(number=w5787) -> (decimal integer string=w5793:string)  [unwired: 1 in]
            n634 = call "S7_Write.vi"("TCP"=w5792, "寄存器类型"=w5800, "DB #"=u16 20, "写入地址"=u32 22, "数据类型"=w5799, "写入数据"=w5787) -> ("TCP"=w5788:refnum<k5>, "error out"=w5789:errorcluster)  [unwired: 7 in, 1 out]
            n635 = Bundle By Name(cluster=w5791, "看门狗"=w5793) -> (w5790:T9)
            n636 = call "S7_Read.vi"("TCP"=w5788, "DB #"=u16 20, "读取长度"=u16 1, "寄存器类型"=w5830, "起始地址"=u32 0, "数据类型"=w5828, "error in"=w5789) -> ("TCP"=w5811:refnum<k5>, "数据"=w5825:u32[], "error out"=w5808:errorcluster)  [unwired: 5 in, 1 out]
            n637 = Index Array(array=w5825, index=0 ("索引")) -> (element=w5823:u32)
            n638 = Number To Boolean Array(number=w5823) -> (Boolean array=w5822:bool[])
            n639 = Index Array(array=w5822, index=2 ("索引")) -> (element=w5812:bool)
            "ST602扫码请求" <- w5812
            n640 = Unbundle By Name(w5790) -> ("扫码超时2"=w5803:string)
            n641 = Not Equal?(x=w5803, y="999") -> (x != y?=w5805:bool)
            n642 = Not(x=w5805) -> (.not. x?=w5806:bool)
            n643 = call <vilib>:"Boolean Crossing PtByPt.vi"("direction"=enum16{"either", "false-true", "true-false"}."false-true", "input"=w5812) -> ("crossing"=w5818:bool)  [unwired: 1 in]
            n644 = call <vilib>:"Boolean Crossing PtByPt.vi"("direction"=enum16{"either", "false-true", "true-false"}."true-false", "input"=w5812) -> ("crossing"=w5817:bool)  [unwired: 1 in]
            n645 = call "已用时间19"("Reset"=w5806) -> ("Time has Elapsed"=w5807:bool)  [unwired: 11 in, 7 out]
            n646 = Insert Into Array(array=bool[] [] ("数组"), index=0 ("索引"), new element #1=w5818, new element #2=w5817) -> (w5814:bool[])
            n647 = Boolean Array To Number(Boolean array=w5814) -> (number=w5813:u32)
            n648 = case shown="2" w5813 {
              tunnel: [cluster{"Data":string[], "State":T1} {"Data"=[], "State"=enum."读数据保存请求2"} ("元素") w5838 w5841] -> w5810
              tunnel: w5802 -> [_ w5839 w5842]
              frame 0, Default {
              }
              frame 1 {
                w5838 = cluster{"Data":string[], "State":T1} {"Data"=[], "State"=enum."读二维码2"} ("元素")
                n649 = Enqueue Element(queue=w5839, element=w5838, timeout in ms (-1)=10 ("超时毫秒(-1)")) -> ()  [unwired: 1 in, 3 out]
              }
              frame 2 {
                w5841 = cluster{"Data":string[], "State":T1} {"Data"=["999"], "State"=enum."扫码回复2"} ("元素")
                n650 = Enqueue Element(queue=w5842, element=w5841, timeout in ms (-1)=10 ("超时毫秒(-1)")) -> ()  [unwired: 1 in, 3 out]
              }
            }
            n651 = case shown="真" w5807 {
              tunnel: w5802 -> [_ w5834]
              frame False {
              }
              frame True {
                n652 = Enqueue Element(queue=w5834, element=cluster{"Data":string[], "State":T1} {"Data"=["999"], "State"=enum."扫码回复2"} ("元素"), timeout in ms (-1)=10 ("超时毫秒(-1)")) -> ()  [unwired: 1 in, 3 out]
              }
            }
          }
          frame "读二维码2" {
            w5858 = u16 0 items=["byte", "word", "Dword"] ("数据类型")
            w5854 = u8 132 items=["I/O (P)"=128, "Input (I)"=129, "Output (Q)"=130, "Bit Memory (M)"=131, "Data (DB)"=132, "Instance Data (DI)"=133, "Local Data (L)"=134, "Predecessor Local Data (VL)"=135] ("寄存器类型")
            n653 = call "S7_Read.vi"("TCP"=w5853, "DB #"=u16 20, "读取长度"=u16 17, "寄存器类型"=w5854, "起始地址"=u32 42, "数据类型"=w5858) -> ("TCP"=w5852:refnum<k5>, "数据"=w5859:u32[], "error out"=w5861:errorcluster)  [unwired: 6 in, 1 out]
            n654 = To Unsigned Word Integer(number=w5859) -> (unsigned 16bit integer=w5860:u16[])
            n655 = call "还原为字符串.vi"("error in (no error)"=w5861, "输入数组"=w5860) -> ("error out"=w5845:errorcluster, "字符串"=w5846:string)  [unwired: 8 in]
            n656 = Match Pattern(string=w5846, regular expression=" " ("正则表达式")) -> (before substring=w5843:string)  [unwired: 1 in, 3 out]
            n657 = flat-sequence {
              tunnel: w5845 -> [w5863]
              tunnel: [w5863] -> w5844
              tunnel: w5843 -> [w5862]
              tunnel: [w5865] -> w5851
              tunnel: w5844 -> [w5864]
              frame #0 {
                "602二维码" <- w5862
              }
              frame #1 {
                n658 = property on="ST602扫码请求(事件)" class="Bool (严格)"(error in=w5864, "Val(Sgnl)"=TRUE ("值(信号)")) -> (error out=w5865:errorcluster)  [unwired: 1 in, 1 out]
              }
            }
          }
          frame "扫码回复2" {
            n659 = Array Size(array=w5875) -> (size(s)=w5876:i32)
            n660 = case shown="3, 默认" w5876 {
              tunnel: w5875 -> [w5878 w5912]
              tunnel: w5874 -> [w5879 w5899]
              tunnel: [w5881 w5890] -> w5873
              tunnel: [w5880 w5889] -> w5872
              tunnel: [w5877 w5888] -> w5867
              frame 1 {
                w5884 = u8 132 items=["I/O (P)"=128, "Input (I)"=129, "Output (Q)"=130, "Bit Memory (M)"=131, "Data (DB)"=132, "Instance Data (DI)"=133, "Local Data (L)"=134, "Predecessor Local Data (VL)"=135] ("寄存器类型")
                w5883 = u16 1 items=["byte", "word", "Dword"] ("数据类型")
                n661 = Index Array(array=w5878) -> (element=w5877:string)  [unwired: 1 in]
                n662 = Decimal String To Number(string=w5877, default (0L)=u32 0 ("默认(0 I32)")) -> (number=w5887:u32)  [unwired: 1 in, 1 out]
                n663 = call "S7_Write.vi"("TCP"=w5879, "寄存器类型"=w5884, "DB #"=u16 20, "写入地址"=u32 14, "数据类型"=w5883, "写入数据"=w5887) -> ("TCP"=w5881:refnum<k5>, "error out"=w5880:errorcluster)  [unwired: 7 in, 1 out]
              }
              frame 3, Default {
                w5902 = u8 132 items=["I/O (P)"=128, "Input (I)"=129, "Output (Q)"=130, "Bit Memory (M)"=131, "Data (DB)"=132, "Instance Data (DI)"=133, "Local Data (L)"=134, "Predecessor Local Data (VL)"=135] ("寄存器类型")
                w5901 = u16 1 items=["byte", "word", "Dword"] ("数据类型")
                w5909 = u8 132 items=["I/O (P)"=128, "Input (I)"=129, "Output (Q)"=130, "Bit Memory (M)"=131, "Data (DB)"=132, "Instance Data (DI)"=133, "Local Data (L)"=134, "Predecessor Local Data (VL)"=135] ("寄存器类型")
                w5910 = u16 1 items=["byte", "word", "Dword"] ("数据类型")
                w5916 = u8 132 items=["I/O (P)"=128, "Input (I)"=129, "Output (Q)"=130, "Bit Memory (M)"=131, "Data (DB)"=132, "Instance Data (DI)"=133, "Local Data (L)"=134, "Predecessor Local Data (VL)"=135] ("寄存器类型")
                w5915 = u16 1 items=["byte", "word", "Dword"] ("数据类型")
                n664 = Index Array(array=w5912) -> (element #1=w5888:string, element #2=w5895:string, element #3=w5894:string)  [unwired: 3 in]
                n665 = Equal?(x=w5894, y="OK") -> (x = y?=w5892:bool)
                n666 = Decimal String To Number(string=w5895, default (0L)=u32 0 ("默认(0 I32)")) -> (number=w5896:u32)  [unwired: 1 in, 1 out]
                n667 = case shown="假" w5892 {
                  tunnel: [u32 2 ("写入数据") u32 1 ("写入数据")] -> w5891
                  frame False {
                  }
                  frame True {
                  }
                }
                n668 = call "S7_Write.vi"("TCP"=w5899, "寄存器类型"=w5916, "DB #"=u16 20, "写入地址"=u32 18, "数据类型"=w5915, "写入数据"=w5896) -> ("TCP"=w5906:refnum<k5>, "error out"=w5907:errorcluster)  [unwired: 7 in, 1 out]
                n669 = call "S7_Write.vi"("TCP"=w5906, "寄存器类型"=w5909, "DB #"=u16 20, "写入地址"=u32 20, "数据类型"=w5910, "写入数据"=w5891, "error in"=w5907) -> ("TCP"=w5898:refnum<k5>, "error out"=w5897:errorcluster)  [unwired: 6 in, 1 out]
                n670 = Decimal String To Number(string=w5888, default (0L)=u32 0 ("默认(0 I32)")) -> (number=w5905:u32)  [unwired: 1 in, 1 out]
                n671 = call "S7_Write.vi"("TCP"=w5898, "寄存器类型"=w5902, "DB #"=u16 20, "写入地址"=u32 14, "数据类型"=w5901, "写入数据"=w5905, "error in"=w5897) -> ("TCP"=w5890:refnum<k5>, "error out"=w5889:errorcluster)  [unwired: 6 in, 1 out]
              }
            }
            "扫码请求回复602" <- w5867
            n672 = Bundle By Name(cluster=w5869, "扫码超时2"=w5867) -> (w5868:T9)
          }
          frame "-- --------------" {
          }
          frame "读数据保存请求2" {
            w5953 = u16 0 items=["byte", "word", "Dword"] ("数据类型")
            w5955 = u8 132 items=["I/O (P)"=128, "Input (I)"=129, "Output (Q)"=130, "Bit Memory (M)"=131, "Data (DB)"=132, "Instance Data (DI)"=133, "Local Data (L)"=134, "Predecessor Local Data (VL)"=135] ("寄存器类型")
            n673 = call "S7_Read.vi"("TCP"=w5936, "DB #"=u16 20, "读取长度"=u16 1, "寄存器类型"=w5955, "起始地址"=u32 0, "数据类型"=w5953) -> ("TCP"=w5935:refnum<k5>, "数据"=w5950:u32[], "error out"=w5934:errorcluster)  [unwired: 6 in, 1 out]
            n674 = Index Array(array=w5950, index=0 ("索引")) -> (element=w5948:u32)
            n675 = Number To Boolean Array(number=w5948) -> (Boolean array=w5947:bool[])
            n676 = Index Array(array=w5947, index=3 ("索引")) -> (element=w5937:bool)
            "ST602数据读取" <- w5937
            n677 = Unbundle By Name(w5926) -> ("数据保存超时2"=w5927:string)
            n678 = Not Equal?(x=w5927, y="999") -> (x != y?=w5929:bool)
            n679 = Not(x=w5929) -> (.not. x?=w5930:bool)
            n680 = call <vilib>:"Boolean Crossing PtByPt.vi"("direction"=enum16{"either", "false-true", "true-false"}."false-true", "input"=w5937) -> ("crossing"=w5940:bool)  [unwired: 1 in]
            n681 = call <vilib>:"Boolean Crossing PtByPt.vi"("direction"=enum16{"either", "false-true", "true-false"}."true-false", "input"=w5937) -> ("crossing"=w5941:bool)  [unwired: 1 in]
            n682 = call "已用时间20"("Reset"=w5930) -> ("Time has Elapsed"=w5931:bool)  [unwired: 11 in, 7 out]
            n683 = Insert Into Array(array=bool[] [] ("数组"), index=0 ("索引"), new element #1=w5940, new element #2=w5941) -> (w5944:bool[])
            n684 = Boolean Array To Number(Boolean array=w5944) -> (number=w5945:u32)
            n685 = case shown="真" w5931 {
              tunnel: w5925 -> [_ w5957]
              frame False {
              }
              frame True {
                n686 = Enqueue Element(queue=w5957, element=cluster{"Data":string[], "State":T1} {"Data"=["999"], "State"=enum."数据保存回复2"} ("元素"), timeout in ms (-1)=10 ("超时毫秒(-1)")) -> ()  [unwired: 1 in, 3 out]
              }
            }
            n687 = case shown="1" w5945 {
              tunnel: [cluster{"Data":string[], "State":T1} {"Data"=[], "State"=enum."看门狗"} ("元素") w5961 w5963] -> w5933
              tunnel: w5925 -> [_ w5962 w5964]
              frame 0, Default {
              }
              frame 1 {
                w5961 = cluster{"Data":string[], "State":T1} {"Data"=[], "State"=enum."读数据2"} ("元素")
                n688 = Enqueue Element(queue=w5962, element=w5961, timeout in ms (-1)=10 ("超时毫秒(-1)")) -> ()  [unwired: 1 in, 3 out]
              }
              frame 2 {
                w5963 = cluster{"Data":string[], "State":T1} {"Data"=["999"], "State"=enum."数据保存回复2"} ("元素")
                n689 = Enqueue Element(queue=w5964, element=w5963, timeout in ms (-1)=10 ("超时毫秒(-1)")) -> ()  [unwired: 1 in, 3 out]
              }
            }
          }
          frame "读数据2" {
            w5990 = u16 1 items=["byte", "word", "Dword"] ("数据类型")
            w5986 = u8 132 items=["I/O (P)"=128, "Input (I)"=129, "Output (Q)"=130, "Bit Memory (M)"=131, "Data (DB)"=132, "Instance Data (DI)"=133, "Local Data (L)"=134, "Predecessor Local Data (VL)"=135] ("寄存器类型")
            n690 = call "S7_Read.vi"("TCP"=w5970, "DB #"=u16 20, "读取长度"=u16 1, "寄存器类型"=w5986, "起始地址"=u32 12, "数据类型"=w5990) -> ("TCP"=w5975:refnum<k5>, "数据"=w5985:u32[], "error out"=w5968:errorcluster)  [unwired: 6 in, 1 out]
            n691 = Index Array(array=w5985) -> (element=w5976:u32)  [unwired: 1 in]
            n692 = Equal?(x=w5976, y=u32 1) -> (x = y?=w5983:bool)
            n693 = case shown="假" w5983 {
              tunnel: ["NG" "OK"] -> w5969
              frame False {
              }
              frame True {
              }
            }
            n694 = Format Date/Time String(time format string (%c)="%Y-%m-%d" ("时间格式字符串(%c)")) -> (date/time string=w5978:string)  [unwired: 2 in]
            n695 = Get Date/Time String() -> (time string=w5977:string)  [unwired: 3 in, 1 out]
            n696 = Insert Into Array(array=string[] [] ("数组"), index=0 ("索引"), new element #1="602" ("新元素/子数组"), new element #2=w5969, new element #3=w5978, new element #4=w5977, new element #5=w5969) -> (w5966:string[])
            n697 = flat-sequence {
              tunnel: w5968 -> [w5992]
              tunnel: [w5992] -> w5967
              tunnel: w5966 -> [w5991]
              tunnel: [w5994] -> w5974
              tunnel: w5967 -> [w5993]
              frame #0 {
                "602读取数据" <- w5991
              }
              frame #1 {
                n698 = property on="ST602数据读取(事件)" class="Bool (严格)"(error in=w5993, "Val(Sgnl)"=TRUE ("值(信号)")) -> (error out=w5994:errorcluster)  [unwired: 1 in, 1 out]
              }
            }
          }
          frame "数据保存回复2" {
            w6011 = u8 132 items=["I/O (P)"=128, "Input (I)"=129, "Output (Q)"=130, "Bit Memory (M)"=131, "Data (DB)"=132, "Instance Data (DI)"=133, "Local Data (L)"=134, "Predecessor Local Data (VL)"=135] ("寄存器类型")
            w6012 = u16 1 items=["byte", "word", "Dword"] ("数据类型")
            n699 = Index Array(array=w6003, index=0 ("索引")) -> (element=w5999:string)
            "数据保存请求回复602" <- w5999
            n700 = Decimal String To Number(string=w5999, default (0L)=u32 0 ("默认(0 I32)")) -> (number=w6007:u32)  [unwired: 1 in, 1 out]
            n701 = call "S7_Write.vi"("TCP"=w6006, "寄存器类型"=w6011, "DB #"=u16 20, "写入地址"=u32 16, "数据类型"=w6012, "写入数据"=w6007) -> ("TCP"=w6005:refnum<k5>, "error out"=w6004:errorcluster)  [unwired: 7 in, 1 out]
            n702 = Bundle By Name(cluster=w6000, "数据保存超时2"=w5999) -> (w5998:T9)
          }
          frame "看门狗" {
            w6022 = "\r" ("正则表达式")
            w6029 = u16 0 items=["byte", "word", "Dword"] ("数据类型")
            w6031 = u8 132 items=["I/O (P)"=128, "Input (I)"=129, "Output (Q)"=130, "Bit Memory (M)"=131, "Data (DB)"=132, "Instance Data (DI)"=133, "Local Data (L)"=134, "Predecessor Local Data (VL)"=135] ("寄存器类型")
            w6053 = u8 132 items=["I/O (P)"=128, "Input (I)"=129, "Output (Q)"=130, "Bit Memory (M)"=131, "Data (DB)"=132, "Instance Data (DI)"=133, "Local Data (L)"=134, "Predecessor Local Data (VL)"=135] ("寄存器类型")
            w6052 = u16 1 items=["byte", "word", "Dword"] ("数据类型")
            n703 = Unbundle By Name(w6041) -> ("看门狗"=w6050:string)
            n704 = Decimal String To Number(string=w6050) -> (number=w6049:i32)  [unwired: 2 in, 1 out]
            n705 = Equal?(x=w6049, y=0) -> (x = y?=w6047:bool)
            n706 = case shown="假" w6047 {
              tunnel: [0 ("y") 1 ("y")] -> w6042
              frame False {
              }
              frame True {
              }
            }
            "60" <- w6042
            n707 = Number To Decimal String(number=w6042) -> (decimal integer string=w6043:string)  [unwired: 1 in]
            n708 = call "S7_Write.vi"("TCP"=w6046, "寄存器类型"=w6053, "DB #"=u16 20, "写入地址"=u32 22, "数据类型"=w6052, "写入数据"=w6042) -> ("TCP"=w6028:refnum<k5>, "error out"=w6027:errorcluster)  [unwired: 7 in, 1 out]
            n709 = Bundle By Name(cluster=w6041, "看门狗"=w6043) -> (w6040:T9)
            n710 = call "S7_Read.vi"("TCP"=w6028, "DB #"=u16 20, "读取长度"=u16 80, "寄存器类型"=w6031, "起始地址"=u32 60, "数据类型"=w6029, "error in"=w6027) -> ("TCP"=w6015:refnum<k5>, "数据"=w6038:u32[], "error out"=w6017:errorcluster)  [unwired: 5 in, 1 out]
            n711 = To Unsigned Word Integer(number=w6038) -> (unsigned 16bit integer=w6039:u16[])
            n712 = call "还原为字符串.vi"("输入数组"=w6039) -> ("字符串"=w6037:string)  [unwired: 9 in, 1 out]
            n713 = for {
              N: 4 -> [_]
              tunnel: w6037 -> [w6071]
              tunnel: [w6070] -> w6036 mode=indexing
              shift-right: [w6066] -> _
              shift-left: 0 ("长度（剩余）") -> [w6068]
              n714 = String Subset(string=w6071, offset (0)=w6068, length (rest)=20 ("长度（剩余）")) -> (substring=w6070:string)
              n715 = Add(x=w6068, y=20) -> (x+y=w6066:i32)
            }
            n716 = Index Array(array=w6036) -> (element #1=w6026:string, element #2=w6025:string, element #3=w6024:string, element #4=w6023:string)  [unwired: 4 in]
            n717 = disable-structure shown="启用" {
              disable-tunnel: w6015 -> [w6055 w6059]
              disable-tunnel: [w6055 w6062] -> w6014
              disable-tunnel: w6017 -> [w6056 w6060]
              disable-tunnel: [w6056 w6061] -> w6016
              frame Disabled {
              }
              frame Enabled {
                w6064 = u8 132 items=["I/O (P)"=128, "Input (I)"=129, "Output (Q)"=130, "Bit Memory (M)"=131, "Data (DB)"=132, "Instance Data (DI)"=133, "Local Data (L)"=134, "Predecessor Local Data (VL)"=135] ("寄存器类型")
                w6058 = u16 1 items=["byte", "word", "Dword"] ("数据类型")
                n718 = local read "80产品型号"() -> (w6057:u32)
                n719 = call "S7_Write.vi"("TCP"=w6059, "寄存器类型"=w6064, "DB #"=u16 20, "写入地址"=u32 140, "数据类型"=w6058, "写入数据"=w6057, "error in"=w6060) -> ("TCP"=w6062:refnum<k5>, "error out"=w6061:errorcluster)  [unwired: 6 in, 1 out]
              }
            }
            n720 = Match Pattern(string=w6026, regular expression=w6022) -> (before substring=→"ST60 Disk Spring 5024300":string)  [unwired: 1 in, 3 out]
